vi "质控参数保存.vi"(7 "section":string="氨氮质控参数", 8 "error in (no error)":errorcluster caption="错误输入（无错误）", 11 "参数":T1) -> (0 "error out":errorcluster caption="错误输出")   [LabVIEW 2016, in "质控单元.lvlib"]
uses:
  <vilib>/Utility/config.llb/Write Key (Double).vi
  <vilib>/Utility/config.llb/NI_LVConfig.lvlib
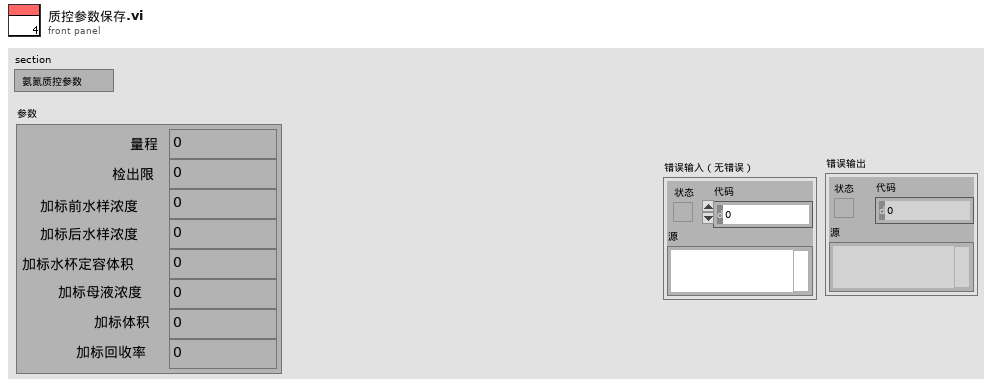
[diagram p1: front panel]
types:
  T1 = cluster{"量程":dbl, "检出限":dbl, "加标前水样浓度":dbl, "加标后水样浓度":dbl, "加标水杯定容体积":dbl, "加标母液浓度":dbl, "加标体积":dbl, "加标回收率":dbl}
  T2 = typedef "NI_LVConfig.lvlib/Config Data RefNum.ctl" = refnum<k1>
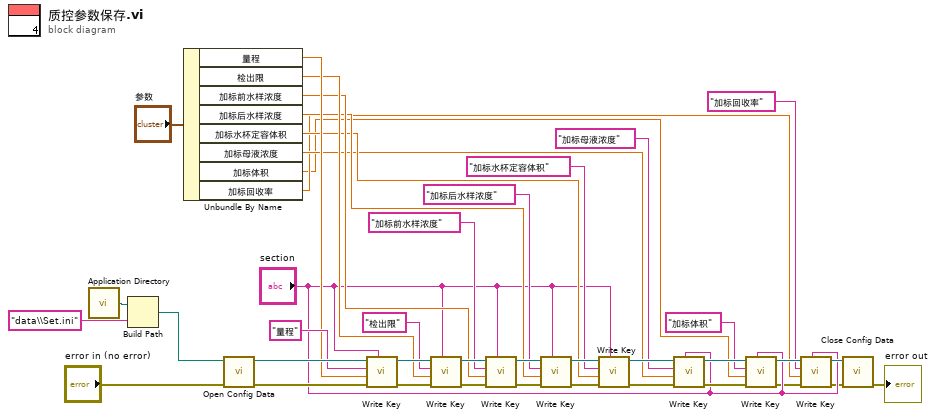
[diagram p0: block diagram]
diagram:
  n1 = call <vilib>:"Application Directory.vi"() -> ("Application Directory"=w39:path)
  n2 = Build Path(base path=w39, name or relative path="data\\Set.ini" ("名称或相对路径")) -> (appended path=w37:path)
  n3 = Unbundle By Name("参数") -> ("量程"=w17:dbl, "检出限"=w16:dbl, "加标前水样浓度"=w15:dbl, "加标后水样浓度"=w14:dbl, "加标水杯定容体积"=w13:dbl, "加标母液浓度"=w12:dbl, "加标体积"=w1:dbl, "加标回收率"=w2:dbl)
  n4 = call <vilib>:"Open Config Data.vi"("error in (no error)"="error in (no error)", "configuration file path"=w37) -> ("error out"=w40:errorcluster, "refnum"=w41:T2)  [unwired: 7 in, 1 out]
  n5 = call-poly <vilib>:"Write Key.vi"("section"="section", "error in (no error)"=w40, "value"=w17, "key"="量程", "refnum"=w41) -> ("error out"=w34:errorcluster, "refnum out"=w35:T2)  [unwired: 4 in, 1 out]
  n6 = call-poly <vilib>:"Write Key.vi"("section"="section", "error in (no error)"=w34, "value"=w16, "key"="检出限", "refnum"=w35) -> ("error out"=w32:errorcluster, "refnum out"=w33:T2)  [unwired: 4 in, 1 out]
  n7 = call-poly <vilib>:"Write Key.vi"("section"="section", "error in (no error)"=w32, "value"=w15, "key"="加标前水样浓度", "refnum"=w33) -> ("error out"=w26:errorcluster, "refnum out"=w27:T2)  [unwired: 4 in, 1 out]
  n8 = call-poly <vilib>:"Write Key.vi"("section"="section", "error in (no error)"=w26, "value"=w14, "key"="加标后水样浓度", "refnum"=w27) -> ("error out"=w29:errorcluster, "refnum out"=w28:T2)  [unwired: 4 in, 1 out]
  n9 = call-poly <vilib>:"Write Key.vi"("section"="section", "error in (no error)"=w29, "value"=w13, "key"="加标水杯定容体积", "refnum"=w28) -> ("error out"=w31:errorcluster, "refnum out"=w30:T2)  [unwired: 4 in, 1 out]
  n10 = call-poly <vilib>:"Write Key.vi"("section"="section", "error in (no error)"=w31, "value"=w12, "key"="加标母液浓度", "refnum"=w30) -> ("error out"=w11:errorcluster, "refnum out"=w10:T2)  [unwired: 4 in, 1 out]
  n11 = call-poly <vilib>:"Write Key.vi"("section"="section", "error in (no error)"=w11, "value"=w1, "key"="加标体积", "refnum"=w10) -> ("error out"=w4:errorcluster, "refnum out"=w9:T2)  [unwired: 4 in, 1 out]
  n12 = call-poly <vilib>:"Write Key.vi"("section"="section", "error in (no error)"=w4, "value"=w2, "key"="加标回收率", "refnum"=w9) -> ("error out"=w3:errorcluster, "refnum out"=w8:T2)  [unwired: 4 in, 1 out]
  n13 = call <vilib>:"Close Config Data.vi"("error in (no error)"=w3, "refnum"=w8) -> ("error out"=→"error out":errorcluster)  [unwired: 8 in, 1 out]
